vi "myRIO_BRig_Host_endExp_folderPath__storeLocation.vi"(10 "input_expPrefix":string) -> (1 "output_folderPath":string)   [LabVIEW 2014]
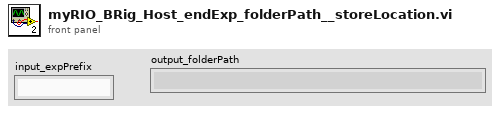
[diagram p1: front panel]
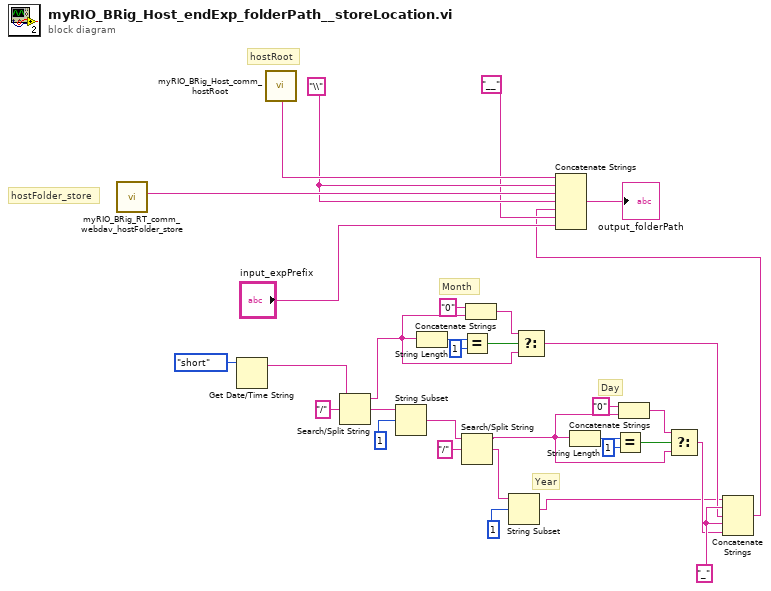
[diagram p0: block diagram]
diagram:
  w11 = "_" ("string")
  w30 = "\\" ("string")
  # "Year"
  # "Day"
  # "Month"
  # "hostFolder_store"
  # "hostRoot"
  n1 = call "myRIO_BRig_RT_comm_webdav_hostFolder_store.vi"() -> ("output_HostFolder"=w32:string)  [unwired: 11 in]
  n2 = Get Date/Time String(date format (0)=enum16{"short", "long", "abbreviated"}."short") -> (date string=w27:string)  [unwired: 2 in, 1 out]
  n3 = call "myRIO_BRig_Host_comm_hostRoot.vi"() -> ("output_hostRoot"=w31:string)  [unwired: 11 in]
  n4 = Search/Split String(string=w27, search string/char (-)="/") -> (substring before match=w19:string, match + rest of string=w7:string)  [unwired: 1 in, 1 out]
  n5 = String Subset(string=w7, offset (0)=1) -> (substring=w5:string)  [unwired: 1 in]
  n6 = String Length(string=w19) -> (length=w23:i32)
  n7 = Equal?(x=w23, y=1) -> (x = y?=w21:bool)
  n8 = Search/Split String(string=w5, search string/char (-)="/") -> (substring before match=w12:string, match + rest of string=w3:string)  [unwired: 1 in, 1 out]
  n9 = Concatenate Strings("0" ("string"), w19) -> (w20:string)
  n10 = String Subset(string=w3, offset (0)=1) -> (substring=w2:string)  [unwired: 1 in]
  n11 = Select(t=w20, s=w21, f=w19) -> (s? t:f=w10:string)
  n12 = String Length(string=w12) -> (length=w17:i32)
  n13 = Equal?(x=w17, y=1) -> (x = y?=w15:bool)
  n14 = Concatenate Strings("0" ("string"), w12) -> (w14:string)
  n15 = Select(t=w14, s=w15, f=w12) -> (s? t:f=w9:string)
  n16 = Concatenate Strings(w2, w11, w10, w11, w9) -> (w8:string)
  n17 = Concatenate Strings(w31, w30, w32, w30, w8, "__" ("string"), "input_expPrefix") -> (→"output_folderPath":string)
